vi "ReplaceOutsideVIs.vi"(8 "error in (no error)":errorcluster, 10 "Non-Library VI[]":string[](array[string]), 11 "TargetDirectory":path) -> (0 "error out":errorcluster)   [LabVIEW 2021, in "Migrator.lvlib"]
uses:
  Migrator.lvlib
  <vilib>/Utility/traverseref.llb/TRef TravTarget.ctl
  <vilib>/Utility/traverseref.llb/VI Scripting - Traverse.lvlib
  Migrator Reusables/Migrator Reusables.lvlib
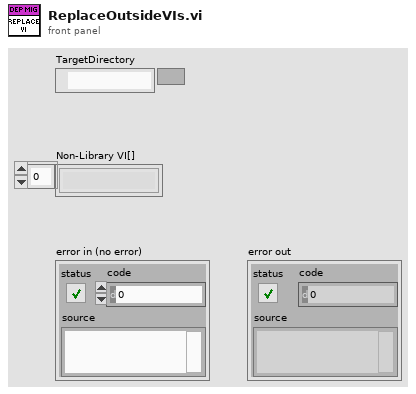
[diagram p1: front panel]
types:
  T1 = typedef "TRef TravTarget.ctl" = enum16{"FP", "BD", "Other"}
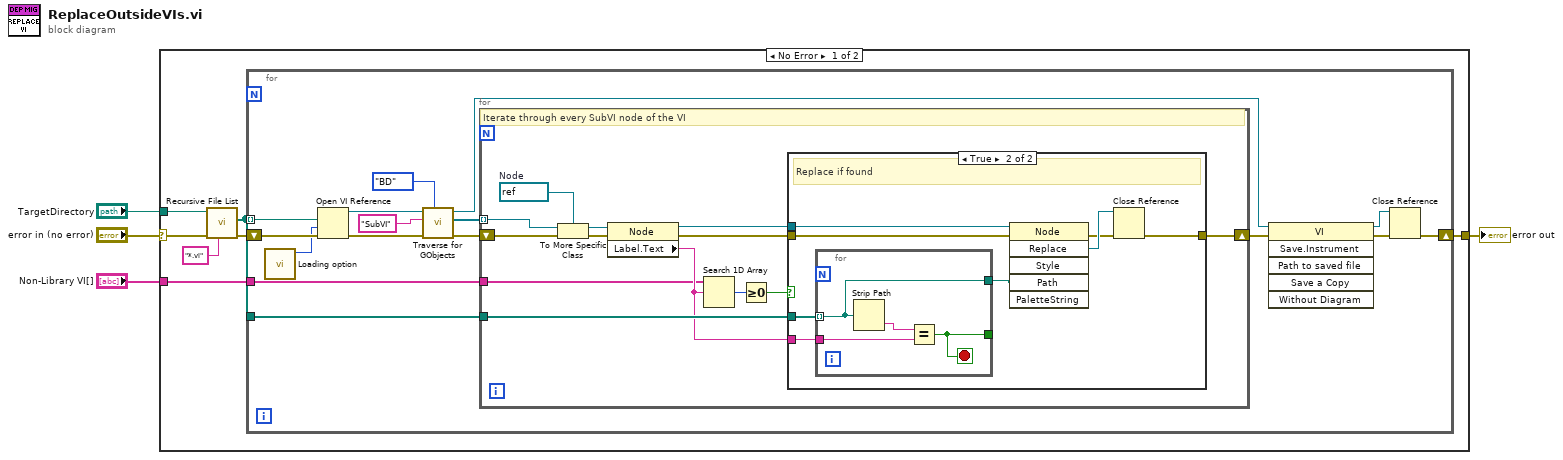
[diagram p0: block diagram]
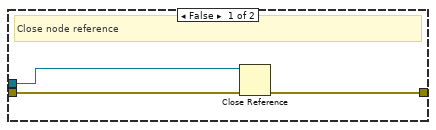
[diagram p2: hidden frame]
diagram:
  n1 = case shown="No Error" "error in (no error)" {
    selector: "error in (no error)" -> [w10 w56]
    tunnel: "Non-Library VI[]" -> [w11 _]
    tunnel: "TargetDirectory" -> [w8 _]
    tunnel: [w6 w56] -> w1
    frame No Error {
      n2 = call <vilib>:"Recursive File List.vi"("pattern"="*.vi", "error in (no error)"=w10, "Folder Path"=w8) -> ("error out"=w9:errorcluster, "All Files in Dir"=w5:path[])  [unwired: 4 in, 3 out]
      n3 = for {
        tunnel: w5 -> [w26]
        tunnel: w11 -> [w25]
        tunnel: w5 -> [w17] mode=indexing
        shift-right: [w18] -> w6
        shift-left: w9 -> [w20]
        n4 = call "Loading option.vi"() -> ("options"=w12:i32)  [unwired: 11 in]
        n5 = Open VI Reference(vi path=w17, options=w12, error in (no error)=w20) -> (vi reference=w16:refnum<vi>, error out=w19:errorcluster)  [unwired: 3 in]
        n6 = call <vilib>:"Traverse for GObjects.vi"("Traverse Target"=TRef_TravTarget."BD", "error in (no error)"=w19, "Class Name"="SubVI" ("name/order"), "VI Refnum"=w16) -> ("error out"=w24:errorcluster, "References"=w27:refnum<vi>[], "dup VI Refnum"=w14:refnum<vi>)  [unwired: 4 in, 1 out]
        n7 = for {
          tunnel: w27 -> [w40] mode=indexing
          shift-right: [w35] -> w23
          shift-left: w24 -> [w39]
          tunnel: w25 -> [w28]
          tunnel: w26 -> [w33]
          w30 = refnum<vi> refnum  # Node
          # "Iterate through every SubVI node of the VI"
          n8 = To More Specific Class(target class=w30, reference=w40, error in=w39) -> (specific class reference=w31:refnum<vi>, error out=w29:errorcluster)
          n9 = property class="Node"(reference=w31, error in=w29) -> (reference out=w36:refnum<vi>, error out=w37:errorcluster, "Label.Text"=w32:string)
          n10 = Search 1D Array(1D array=w28, element=w32) -> (index of element=w38:i32)  [unwired: 1 in]
          n11 = Greater Or Equal To 0?(x=w38) -> (x >= 0?=w34:bool)
          n12 = case shown="True" w34 {
            tunnel: w37 -> [w43 w51]
            tunnel: w36 -> [w42 w50]
            tunnel: [w41 w44] -> w35
            tunnel: w33 -> [_ w49]
            tunnel: w32 -> [_ w48]
            frame False {
              # "Close node reference"
              n13 = Close Reference(reference=w42, error in (no error)=w43) -> (error out=w41:errorcluster)
            }
            frame True {
              # "Replace if found"
              n14 = for {
                tunnel: w49 -> [w53] mode=indexing
                tunnel: w48 -> [w54]
                tunnel: [w53] -> w47
                tunnel: [w52] -> _
                stop <- w52 stop-if-true
                n15 = Strip Path(path=w53) -> (name=w55:string)  [unwired: 1 out]
                n16 = Equal?(x=w55, y=w54) -> (x = y?=w52:bool)
              }
              n17 = invoke class="Node" method="Replace"(reference=w50, error in=w51, "Path"=w47) -> (error out=w45:errorcluster, "Replace"=w46:refnum<vi>)  [unwired: 3 in, 4 out]
              n18 = Close Reference(reference=w46, error in (no error)=w45) -> (error out=w44:errorcluster)
            }
          }
        }
        n19 = invoke class="VI" method="Save.Instrument"(reference=w14, error in=w23) -> (reference out=w13:refnum<vi>, error out=w15:errorcluster)  [unwired: 4 in, 4 out]
        n20 = Close Reference(reference=w13, error in (no error)=w15) -> (error out=w18:errorcluster)
      }
    }
    frame Error {
    }
  }
  "error out" <- w1
